vi "main_interface.vi"() -> ()   [LabVIEW 2024]
uses:
  <vilib>/numeric/Random Number (Range) U64.vi
  <vilib>/numeric/sub_Random U32.vi
panel:
  out "Turn count":u8
  out "消除數":u16
  out "分數":u32
  out "blocks left":u8
  out "Preview":picture
  in  "Next block":bool
  out "cur block":u8
  out "buf block type":u8[](array[numeric])
  out "rng array":u8[][](array[numeric])
  out "待放置方塊":picture
  in  "direction":enum16{"up", "right", "down", "left"}(ring)
  out "Plate array":u8[][](array[numeric])
  in  "choose_block":u16
  in  "stop":bool
  out "plate":picture
  in  "Turn Block":bool
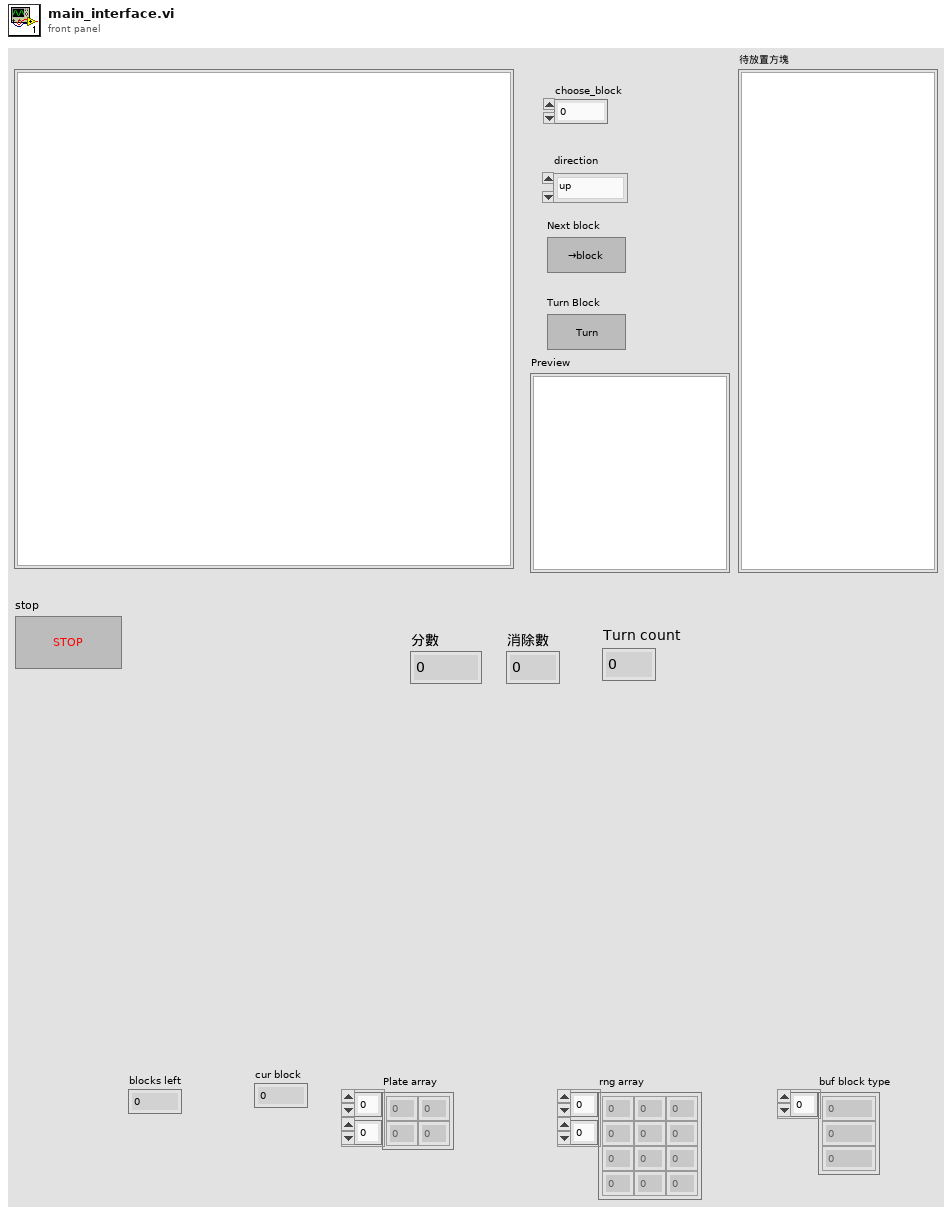
[diagram p1: front panel]
types:
  T1 = typedef "LVPoint32TypeDef.ctl" = cluster{"Horizontal":i32, "Vertical":i32}
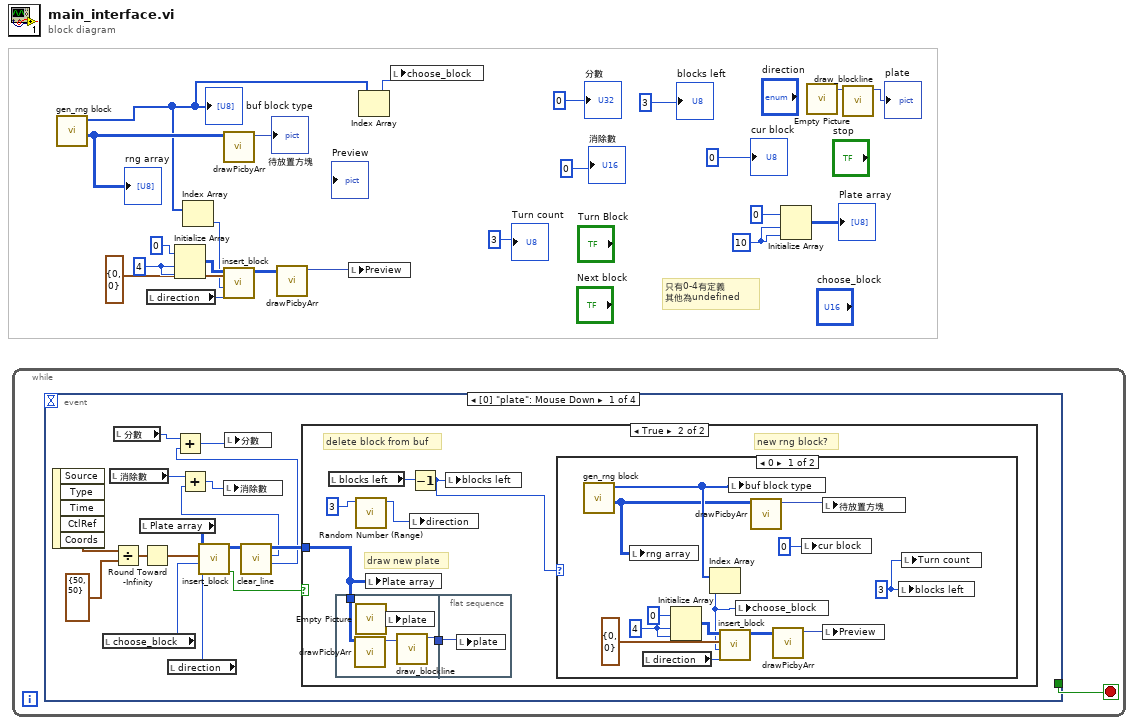
[diagram p0: block diagram]
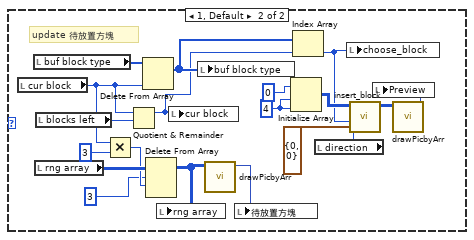
[diagram p3: hidden frame]
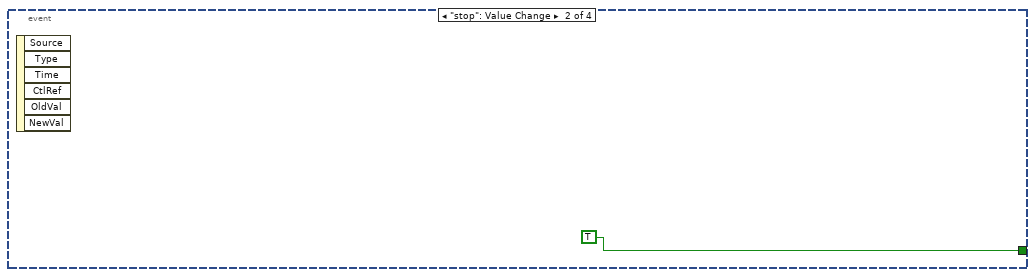
[diagram p4: hidden frame]
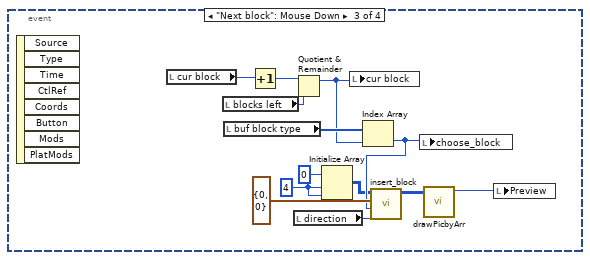
[diagram p5: hidden frame]
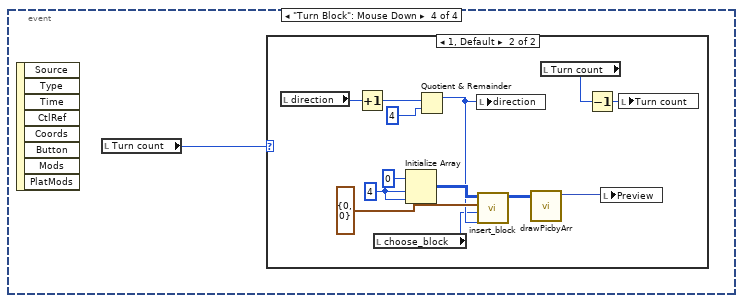
[diagram p6: hidden frame]
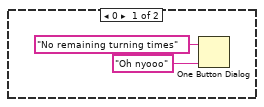
[diagram p7: hidden frame]
diagram:
  w16 = 4 ("dimension size")
  w20 = 10
  # "只有0-4有定義\n其他為undefined"
  n1 = while {
    stop <- w23 stop-if-true
    n2 = event shown="[0] \"plate\": Mouse Down" {
      selector: _ -> [_ _ _ _]
      dyn-events: _ -> [_ _ _ _]
      timeout: _ -> [_ _ _ _]
      tunnel: [_ TRUE _ _] -> w23
      event "plate": Mouse Down {
        n3 = event-data() -> ("Coords"=w37:T1)  [unwired: 1 in, 4 out]
        n4 = local read "choose_block"() -> (w36:u16)
        n5 = local read "消除數"() -> (w29:u16)
        n6 = Divide(x=w37, y=cluster{"Horizontal":u16, "Vertical":u16} {"Horizontal"=50, "Vertical"=50}) -> (x/y=w39:cluster{"Horizontal":dbl, "Vertical":dbl})
        n7 = local read "分數"() -> (w28:u32)
        n8 = local read "Plate array"() -> (w35:u8[][])
        n9 = Round Toward -Infinity(1:w39) -> (0:w33:cluster{"Horizontal":dbl, "Vertical":dbl})
        n10 = local read "direction"() -> (w32:enum16{"up", "right", "down", "left"})
        n11 = call "insert_block.vi"("direction"=w32, "block_type"=w36, "position"=w33, "plate arr"=w35) -> ("valid?"=w34:bool, "return plate"=w31:u8[][])  [unwired: 6 in]
        n12 = call "clear_line.vi"("Array in"=w31) -> ("得分"=w26:u32, "消除數"=w27:u8, "Array out"=w30:u8[][])  [unwired: 8 in]
        n13 = Add(x=w28, y=w26) -> (x+y=w25:u32)
        n14 = Add(x=w29, y=w27) -> (x+y=w24:u16)
        n15 = local write "消除數"(w24) -> ()
        n16 = local write "分數"(w25) -> ()
        n17 = case shown="True" w34 {
          tunnel: w30 -> [_ w45]
          frame False {
          }
          frame True {
            # "new rng block?"
            # "delete block from buf"
            # "draw new plate"
            n18 = local read "blocks left"() -> (w43:u8)
            n19 = flat-sequence {
              tunnel: w45 -> [w81]
              tunnel: [w78] -> w44
              tunnel: w44 -> [w82]
              frame #0 {
                n20 = call "drawPicbyArr.vi"("Array"=w81) -> ("2D Picture"=w79:picture)  [unwired: 10 in]
                n21 = call "Empty Picture"() -> ("empty picture"=w80:picture)
                n22 = local write "plate"(w80) -> ()
                n23 = call "draw_blockline.vi"("picture in"=w79) -> ("picture out"=w78:picture)  [unwired: 10 in]
              }
              frame #1 {
                n24 = local write "plate"(w82) -> ()
              }
            }
            n25 = call-poly <vilib>:"Random Number (Range).vi"("upper bound (100)"=u64 3 ("lower bound (0)")) -> ("number"=w41:u64)  [unwired: 10 in]
            n26 = local write "Plate array"(w45) -> ()
            n27 = Decrement(x=w43) -> (x-1=w42:u8)
            n28 = local write "direction"(w41) -> ()
            n29 = local write "blocks left"(w42) -> ()
            n30 = case shown="0" w42 {
              frame 0 {
                w46 = u8 3 ("blocks left")
                w53 = 4 ("dimension size")
                n31 = call "gen_rng block.vi"() -> ("display arr"=w49:u8[][], "Random block"=w51:u8[])  [unwired: 10 in]
                n32 = local write "rng array"(w49) -> ()
                n33 = local read "direction"() -> (w56:enum16{"up", "right", "down", "left"})
                n34 = Initialize Array(u8 0 ("element"), w53, w53) -> (w52:u8[][])
                n35 = Index Array(array=w51) -> (element=w48:u8)  [unwired: 1 in]
                n36 = call "insert_block.vi"("direction"=w56, "block_type"=w48, "position"=cluster{"x":u8, "y":u8} {"x"=0, "y"=0}, "plate arr"=w52) -> ("return plate"=w58:u8[][])  [unwired: 6 in, 1 out]
                n37 = local write "buf block type"(w51) -> ()
                n38 = local write "choose_block"(w48) -> ()
                n39 = call "drawPicbyArr.vi"("Array"=w49) -> ("2D Picture"=w50:picture)  [unwired: 10 in]
                n40 = call "drawPicbyArr.vi"("Array"=w58) -> ("2D Picture"=w57:picture)  [unwired: 10 in]
                n41 = local write "cur block"(u8 0 ("cur block")) -> ()
                n42 = local write "待放置方塊"(w50) -> ()
                n43 = local write "Preview"(w57) -> ()
                n44 = local write "blocks left"(w46) -> ()
                n45 = local write "Turn count"(w46) -> ()
              }
              frame 1, Default {
                w65 = 4 ("dimension size")
                # "update 待放置方塊"
                n46 = local read "cur block"() -> (w61:u8)
                n47 = local read "buf block type"() -> (w77:u8[])
                n48 = local read "rng array"() -> (w76:u8[][])
                n49 = local read "blocks left"() -> (w59:u8)
                n50 = Multiply(x=w61, y=u8 3) -> (x*y=w74:u8)
                n51 = Quotient & Remainder(x=w61, y=w59) -> (x-y*floor(x/y)=w60:u8)  [unwired: 1 out]
                n52 = Delete From Array(array=w77, index=w61) -> (array with subset deleted=w63:u8[])  [unwired: 1 in, 1 out]
                n53 = Delete From Array(array=w76, length=3, index (row)=w74) -> (array with subset deleted=w72:u8[][])  [unwired: 1 in, 1 out]
                n54 = local write "rng array"(w72) -> ()
                n55 = local write "cur block"(w60) -> ()
                n56 = local write "buf block type"(w63) -> ()
                n57 = call "drawPicbyArr.vi"("Array"=w72) -> ("2D Picture"=w71:picture)  [unwired: 10 in]
                n58 = local write "待放置方塊"(w71) -> ()
                n59 = Initialize Array(u8 0 ("element"), w65, w65) -> (w67:u8[][])
                n60 = Index Array(array=w63, index=w60) -> (element=w62:u8)
                n61 = local read "direction"() -> (w68:enum16{"up", "right", "down", "left"})
                n62 = local write "choose_block"(w62) -> ()
                n63 = call "insert_block.vi"("direction"=w68, "block_type"=w62, "position"=cluster{"x":u8, "y":u8} {"x"=0, "y"=0}, "plate arr"=w67) -> ("return plate"=w70:u8[][])  [unwired: 6 in, 1 out]
                n64 = call "drawPicbyArr.vi"("Array"=w70) -> ("2D Picture"=w69:picture)  [unwired: 10 in]
                n65 = local write "Preview"(w69) -> ()
              }
            }
          }
        }
      }
      event "stop": Value Change {
        n66 = event-data() -> ()  [unwired: 1 in, 6 out]
      }
      event "Next block": Mouse Down {
        w86 = 4 ("dimension size")
        n67 = event-data() -> ()  [unwired: 1 in, 8 out]
        n68 = local read "cur block"() -> (w96:u8)
        n69 = local read "blocks left"() -> (w84:u8)
        n70 = local read "buf block type"() -> (w94:u8[])
        n71 = Increment(x=w96) -> (x+1=w95:u8)
        n72 = Quotient & Remainder(x=w95, y=w84) -> (x-y*floor(x/y)=w93:u8)  [unwired: 1 out]
        n73 = local read "direction"() -> (w90:enum16{"up", "right", "down", "left"})
        n74 = Initialize Array(u8 0 ("element"), w86, w86) -> (w85:u8[][])
        n75 = local write "cur block"(w93) -> ()
        n76 = Index Array(array=w94, index=w93) -> (element=w88:u8)
        n77 = call "insert_block.vi"("direction"=w90, "block_type"=w88, "position"=cluster{"x":u8, "y":u8} {"x"=0, "y"=0}, "plate arr"=w85) -> ("return plate"=w92:u8[][])  [unwired: 6 in, 1 out]
        n78 = local write "choose_block"(w88) -> ()
        n79 = call "drawPicbyArr.vi"("Array"=w92) -> ("2D Picture"=w91:picture)  [unwired: 10 in]
        n80 = local write "Preview"(w91) -> ()
      }
      event "Turn Block": Mouse Down {
        n81 = event-data() -> ()  [unwired: 1 in, 8 out]
        n82 = local read "Turn count"() -> (w97:u8)
        n83 = case shown="1, Default" w97 {
          frame 0 {
            n84 = One Button Dialog(message="No remaining turning times", button name ("OK")="Oh nyooo") -> ()  [unwired: 1 out]
          }
          frame 1, Default {
            w108 = 4 ("dimension size")
            n85 = local read "direction"() -> (w106:enum16{"up", "right", "down", "left"})
            n86 = Increment(x=w106) -> (x+1=w105:enum16{"up", "right", "down", "left"})
            n87 = local read "choose_block"() -> (w102:u16)
            n88 = Initialize Array(u8 0 ("element"), w108, w108) -> (w110:u8[][])
            n89 = Quotient & Remainder(x=w105, y=4) -> (x-y*floor(x/y)=w103:i32)  [unwired: 1 out]
            n90 = local write "direction"(w103) -> ()
            n91 = call "insert_block.vi"("direction"=w103, "block_type"=w102, "position"=cluster{"x":u8, "y":u8} {"x"=0, "y"=0}, "plate arr"=w110) -> ("return plate"=w112:u8[][])  [unwired: 6 in, 1 out]
            n92 = call "drawPicbyArr.vi"("Array"=w112) -> ("2D Picture"=w111:picture)  [unwired: 10 in]
            n93 = local read "Turn count"() -> (w101:u8)
            n94 = Decrement(x=w101) -> (x-1=w100:u8)
            n95 = local write "Preview"(w111) -> ()
            n96 = local write "Turn count"(w100) -> ()
          }
        }
      }
    }
  }
  n97 = call "gen_rng block.vi"() -> ("display arr"=w18:u8[][], "Random block"=w8:u8[])  [unwired: 10 in]
  "rng array" <- w18
  "buf block type" <- w8
  n98 = local read "direction"() -> (w13:enum16{"up", "right", "down", "left"})
  n99 = Initialize Array(u8 0 ("element"), w16, w16) -> (w17:u8[][])
  n100 = Index Array(array=w8) -> (element=w10:u8)  [unwired: 1 in]
  n101 = call "drawPicbyArr.vi"("Array"=w18) -> ("2D Picture"=→"待放置方塊":picture)  [unwired: 10 in]
  n102 = call "insert_block.vi"("direction"=w13, "block_type"=w10, "position"=cluster{"x":u8, "y":u8} {"x"=0, "y"=0}, "plate arr"=w17) -> ("return plate"=w11:u8[][])  [unwired: 6 in, 1 out]
  n103 = call "drawPicbyArr.vi"("Array"=w11) -> ("2D Picture"=w12:picture)  [unwired: 10 in]
  n104 = local write "Preview"(w12) -> ()
  n105 = Index Array(array=w8) -> (element=w7:u8)  [unwired: 1 in]
  n106 = local write "choose_block"(w7) -> ()
  n107 = Initialize Array(u8 0 ("element"), w20, w20) -> (→"Plate array":u8[][])
  n108 = call "Empty Picture"() -> ("empty picture"=w5:picture)
  n109 = call "draw_blockline.vi"("picture in"=w5) -> ("picture out"=→"plate":picture)  [unwired: 10 in]
  "cur block" <- 0
  "blocks left" <- u8 3 ("blocks left")
  "分數" <- 0
  "消除數" <- u16 0 ("消除數")
  "Turn count" <- 3
